vi "Lab Panel V6.00.vi"() -> ()   [LabVIEW 2017] (continued)
                        n2201 = local read "AI data 1"() -> (w3889:waveform(dbl)[])
                        n2202 = local read "AI data 2"() -> (w3886:waveform(dbl)[])
                        n2203 = local read "AI Error"() -> (w3888:errorcluster[])
                        n2204 = call "sub vi - Read Analog All v9.5.vi"("data 0"=w3890, "data 1"=w3889, "data 2"=w3886, "AI Error"=w3888) -> ("Lab05 -1 Offset I"=→"Lab05 -1 Offset I":dbl, "array GRAPH"=w3898:dynamicdata[], "LAB01"=w3897:T33, "LAB02"=w3896:T34, "LAB03"=w3895:T35, "LAB04"=w3894:T36, "deg C"=w3892:dbl, "USB Error"=w3891:bool[], "LAB05"=w3893:T17)  [unwired: 3 in]
                        "LAB05" <- w3893
                        n2205 = local read "AI loop time"() -> (w3887:dbl)
                      }
                    }
                  }
                  frame True {
                    # "simulate"
                    n2206 = local read "ON amps"() -> (w3902:dbl)
                    n2207 = local read "OFF amps"() -> (w3903:dbl)
                    n2208 = local read "VOLTS"() -> (w3906:dbl)
                    n2209 = local read "PF"() -> (w3905:dbl)
                    n2210 = Select(t=w3902, s=w3908, f=w3903) -> (s? t:f=w3907:dbl)
                    n2211 = Bundle("OFF amps"=w3907, "VOLTS"=w3906, "PF"=w3905, "OFF amps"=w3907, "VOLTS"=w3906, "PF"=w3905) -> (w3904:T37)  [unwired: 1 in]
                  }
                }
                n2212 = local read "DAQ Simulate"() -> (w3861:bool)
                n2213 = stacked-sequence {
                  seq-local: [w3912 _ _ _ _ _ _ _] -> [_ _ _ _ _ _ _ _]
                  seq-local: [w3911 _ _ _ _ _ _ _] -> [_ _ _ _ _ _ _ _]
                  seq-local: [w3910 _ _ _ _ _ _ _] -> [_ _ _ _ _ _ _ w4137]
                  tunnel: w3868 -> [_ w3964 _ _ _ _ _ _]
                  tunnel: w3867 -> [_ _ w3997 _ _ _ _ _]
                  tunnel: w3866 -> [_ _ _ w4031 _ _ _ _]
                  tunnel: w3865 -> [_ _ _ _ w4065 _ _ _]
                  tunnel: w3864 -> [_ _ _ _ _ w4099 _ _]
                  tunnel: w3863 -> [_ _ _ _ _ _ w4134 _]
                  tunnel: w3861 -> [_ _ w3996 w4030 w4064 w4098 w4133 w4139]
                  tunnel: T15 {"1  (A) cal"=1.0, "1 (V) cal"=1.0, "1 (PF) cal"=1.0, "1 (TL) cal"=1.0, "1 (TN) cal"=1.0, "2 (A) cal"=1.0, "2 (V) cal"=1.0, "2 (PF) cal"=1.0, "2 (TL) cal"=1.0, "2 (TN) cal"=1.0} ("CAL LAB01") -> [_ _ w3995 w4029 w4063 w4097 w4132 _]
                  tunnel: w3858 -> [_ _ _ _ _ _ _ w4138]
                  tunnel: w3857 -> [w3915 _ _ _ _ _ _ _]
                  tunnel: w3855 -> [_ w3943 _ _ _ _ _ _]
                  frame #0 {
                    # "Count DAQ errors. If greater than 10 do USB reset"
                    n2214 = Index Array(array=w3915, index=2) -> (element=w3910:bool)
                    n2215 = Index Array(array=w3915, index=1) -> (element=w3911:bool)
                    n2216 = Index Array(array=w3915, index=0) -> (element=w3912:bool)
                    n2217 = local write "Error USB #2"(w3910) -> ()
                    n2218 = local write "Error USB #0"(w3912) -> ()
                    n2219 = local write "Error USB #1"(w3911) -> ()
                    n2220 = stacked-sequence {
                      tunnel: w3912 -> [w3919 _ _ _]
                      tunnel: w3911 -> [_ w3924 _ _]
                      tunnel: 0 -> [w3918 w3923 w3928 _]
                      tunnel: w3910 -> [_ _ w3929 _]
                      frame #0 {
                        n2221 = case shown="True" w3919 {
                          tunnel: w3918 -> [w3920 _]
                          frame False {
                            n2222 = local write "Er USB#0"(w3920) -> ()
                          }
                          frame True {
                            n2223 = local read "Er USB#0"() -> (w3922:dbl)
                            n2224 = Increment(x=w3922) -> (x+1=→"Er USB#0":dbl)
                          }
                        }
                      }
                      frame #1 {
                        n2225 = case shown="True" w3924 {
                          tunnel: w3923 -> [w3925 _]
                          frame False {
                            n2226 = local write "Er USB#1"(w3925) -> ()
                          }
                          frame True {
                            n2227 = local read "Er USB#1"() -> (w3927:dbl)
                            n2228 = Increment(x=w3927) -> (x+1=→"Er USB#1":dbl)
                          }
                        }
                      }
                      frame #2 {
                        n2229 = case shown="True" w3929 {
                          tunnel: w3928 -> [w3930 _]
                          frame False {
                            n2230 = local write "Er USB#2"(w3930) -> ()
                          }
                          frame True {
                            n2231 = local read "Er USB#2"() -> (w3932:dbl)
                            n2232 = Increment(x=w3932) -> (x+1=→"Er USB#2":dbl)
                          }
                        }
                      }
                      frame #3 {
                        w3938 = 10
                        n2233 = local read "Er USB#2"() -> (w3939:dbl)
                        n2234 = local read "Er USB#0"() -> (w3941:dbl)
                        n2235 = local read "Er USB#1"() -> (w3940:dbl)
                        n2236 = Greater Or Equal?(x=w3941, y=w3938) -> (x >= y?=w3936:bool)
                        n2237 = Greater Or Equal?(x=w3940, y=w3938) -> (x >= y?=w3935:bool)
                        n2238 = Greater Or Equal?(x=w3939, y=w3938) -> (x >= y?=w3934:bool)
                        n2239 = Or(x=w3936, y=w3935) -> (x .or. y?=w3937:bool)
                        n2240 = Or(x=w3937, y=w3934) -> (x .or. y?=w3933:bool)
                        "Analog error" <- w3933
                        n2241 = case shown="False" w3933 {
                          frame False {
                            n2242 = call "Less Simple Error Handler.vi"("message"="Error count exceeded") -> ()  [unwired: 5 in]
                          }
                          frame True {
                          }
                        }
                      }
                    }
                  }
                  frame #1 {
                    # "display graph data on ADM page"
                    n2243 = local write "AI loop time"(w3943) -> ()
                    n2244 = local write "AI"(TRUE) -> ()
                    n2245 = Index Array(array=w3964, index=6) -> (element=→"LAB04-1 (GRAPH)":dynamicdata)
                    n2246 = Index Array(array=w3964, index=7) -> (element=→"LAB04-2 (GRAPH)":dynamicdata)
                    n2247 = Index Array(array=w3964, index=9) -> (element=→"LAB05-2 (GRAPH)":dynamicdata)
                    n2248 = Index Array(array=w3964, index=8) -> (element=→"LAB05-1 (GRAPH)":dynamicdata)
                    n2249 = Index Array(array=w3964, index=5) -> (element=→"LAB03-2 (GRAPH)":dynamicdata)
                    n2250 = Index Array(array=w3964, index=0) -> (element=→"LAB01-1 (GRAPH)":dynamicdata)
                    n2251 = Index Array(array=w3964, index=1) -> (element=→"LAB01-2 (GRAPH)":dynamicdata)
                    n2252 = Index Array(array=w3964, index=2) -> (element=→"LAB02-1 (GRAPH)":dynamicdata)
                    n2253 = Index Array(array=w3964, index=3) -> (element=→"LAB02-2 (GRAPH)":dynamicdata)
                    n2254 = Index Array(array=w3964, index=4) -> (element=→"LAB03-1 (GRAPH)":dynamicdata)
                  }
                  frame #2 {
                    n2255 = case shown="False" w3996 {
                      tunnel: [w3998 w3999] -> w3994
                      tunnel: w3995 -> [_ w3999]
                      frame False {
                        n2256 = local read "CAL LAB01"() -> (w3998:T15)
                      }
                      frame True {
                      }
                    }
                    n2257 = Unbundle By Name(w3997) -> ("OFF amps"=w3993:dbl, "VOLTS"=w3992:dbl, "PF"=w3991:dbl, "OFF amps"=w3990:dbl, "VOLTS"=w3989:dbl, "PF"=w3988:dbl)
                    n2258 = Unbundle By Name(w3994) -> ("1  (A) cal"=w3987:dbl, "1 (V) cal"=w3986:dbl, "1 (PF) cal"=w3985:dbl, "2 (A) cal"=w3984:dbl, "2 (V) cal"=w3983:dbl, "2 (PF) cal"=w3982:dbl)  [unwired: 4 out]
                    n2259 = Multiply(x=w3993, y=w3987) -> (x*y=w3979:dbl)
                    n2260 = Multiply(x=w3992, y=w3986) -> (x*y=w3978:dbl)
                    n2261 = Multiply(x=w3991, y=w3985) -> (x*y=w3973:dbl)
                    n2262 = Multiply(x=w3990, y=w3984) -> (x*y=w3976:dbl)
                    n2263 = Multiply(x=w3989, y=w3983) -> (x*y=w3975:dbl)
                    n2264 = Multiply(x=w3988, y=w3982) -> (x*y=w3969:dbl)
                    n2265 = local read "SIG LAB01-2"() -> (w3980:T2)
                    n2266 = call "Check for valid PF.vi"("PF In"=w3973, "VOLTS"=w3978, "Current"=w3979) -> ("PF Out"=w3971:dbl, "V Out"=w3972:dbl, "I Out"=w3977:dbl)  [unwired: 6 in]
                    n2267 = call "Check for valid PF.vi"("PF In"=w3969, "VOLTS"=w3975, "Current"=w3976) -> ("PF Out"=w3968:dbl, "V Out"=w3970:dbl, "I Out"=w3974:dbl)  [unwired: 6 in]
                    n2268 = local read "SIG LAB01-1"() -> (w3981:T2)
                    n2269 = Bundle By Name(cluster=w3981, "AMPS"=w3977, "VOLTS"=w3972, "PF"=w3971) -> (w3967:T2)
                    "SIG LAB01-1" <- w3967
                    n2270 = Bundle By Name(cluster=w3980, "AMPS"=w3974, "VOLTS"=w3970, "PF"=w3968) -> (w3966:T2)
                    "SIG LAB01-2" <- w3966
                    n2271 = global write "Global display 1.vi" "SIG LAB01-2"(w3966) -> ()
                    n2272 = global write "Global display 1.vi" "SIG LAB01-1"(w3967) -> ()
                  }
                  frame #3 {
                    n2273 = Unbundle By Name(w4031) -> ("OFF amps"=w4027:dbl, "VOLTS"=w4026:dbl, "PF"=w4025:dbl, "OFF amps"=w4024:dbl, "VOLTS"=w4023:dbl, "PF"=w4022:dbl)
                    n2274 = case shown="True" w4030 {
                      tunnel: [w4032 w4033] -> w4028
                      tunnel: w4029 -> [_ w4033]
                      frame False {
                        n2275 = local read "CAL LAB02"() -> (w4032:T16)
                      }
                      frame True {
                      }
                    }
                    n2276 = Unbundle By Name(w4028) -> ("1  (A) cal"=w4021:dbl, "1 (V) cal"=w4020:dbl, "1 (PF) cal"=w4019:dbl, "2 (A) cal"=w4018:dbl, "2 (V) cal"=w4017:dbl, "2 (PF) cal"=w4016:dbl)  [unwired: 4 out]
                    n2277 = Multiply(x=w4027, y=w4021) -> (x*y=w4012:dbl)
                    n2278 = Multiply(x=w4026, y=w4020) -> (x*y=w4011:dbl)
                    n2279 = Multiply(x=w4025, y=w4019) -> (x*y=w4004:dbl)
                    n2280 = Multiply(x=w4024, y=w4018) -> (x*y=w4009:dbl)
                    n2281 = Multiply(x=w4023, y=w4017) -> (x*y=w4008:dbl)
                    n2282 = Multiply(x=w4022, y=w4016) -> (x*y=w4003:dbl)
                    n2283 = local read "SIG LAB02-2"() -> (w4014:T2)
                    n2284 = call "Check for valid PF.vi"("PF In"=w4004, "VOLTS"=w4011, "Current"=w4012) -> ("PF Out"=w4006:dbl, "V Out"=w4005:dbl, "I Out"=w4010:dbl)  [unwired: 6 in]
                    n2285 = call "Check for valid PF.vi"("PF In"=w4003, "VOLTS"=w4008, "Current"=w4009) -> ("PF Out"=w4001:dbl, "V Out"=w4002:dbl, "I Out"=w4007:dbl)  [unwired: 6 in]
                    n2286 = local read "SIG LAB02-1"() -> (w4015:T2)
                    n2287 = Bundle By Name(cluster=w4015, "AMPS"=w4010, "VOLTS"=w4005, "PF"=w4006) -> (→"SIG LAB02-1" →"SIG LAB02-2":T2)
                    n2288 = Bundle By Name(cluster=w4014, "AMPS"=w4007, "VOLTS"=w4002, "PF"=w4001) -> (w4013:T2)
                    n2289 = local write "SIG LAB02-2"(w4013) -> ()
                    n2290 = global write "Global display 1.vi" "SIG LAB02-2"(w4013) -> ()
                  }
                  frame #4 {
                    n2291 = Unbundle By Name(w4065) -> ("OFF amps"=w4061:dbl, "VOLTS"=w4060:dbl, "PF"=w4059:dbl, "OFF amps"=w4058:dbl, "VOLTS"=w4057:dbl, "PF"=w4056:dbl)
                    n2292 = case shown="False" w4064 {
                      tunnel: [w4066 w4067] -> w4062
                      tunnel: w4063 -> [_ w4067]
                      frame False {
                        n2293 = local read "CAL LAB03"() -> (w4066:T15)
                      }
                      frame True {
                      }
                    }
                    n2294 = Unbundle By Name(w4062) -> ("1  (A) cal"=w4055:dbl, "1 (V) cal"=w4054:dbl, "1 (PF) cal"=w4053:dbl, "2 (A) cal"=w4052:dbl, "2 (V) cal"=w4051:dbl, "2 (PF) cal"=w4050:dbl)  [unwired: 4 out]
                    n2295 = Multiply(x=w4061, y=w4055) -> (x*y=w4047:dbl)
                    n2296 = Multiply(x=w4060, y=w4054) -> (x*y=w4046:dbl)
                    n2297 = Multiply(x=w4059, y=w4053) -> (x*y=w4041:dbl)
                    n2298 = Multiply(x=w4058, y=w4052) -> (x*y=w4044:dbl)
                    n2299 = Multiply(x=w4057, y=w4051) -> (x*y=w4043:dbl)
                    n2300 = Multiply(x=w4056, y=w4050) -> (x*y=w4040:dbl)
                    n2301 = call "Check for valid PF.vi"("PF In"=w4041, "VOLTS"=w4046, "Current"=w4047) -> ("PF Out"=w4036:dbl, "V Out"=w4037:dbl, "I Out"=w4045:dbl)  [unwired: 6 in]
                    n2302 = call "Check for valid PF.vi"("PF In"=w4040, "VOLTS"=w4043, "Current"=w4044) -> ("PF Out"=w4039:dbl, "V Out"=w4038:dbl, "I Out"=w4042:dbl)  [unwired: 6 in]
                    n2303 = local read "SIG LAB03-1"() -> (w4049:T2)
                    n2304 = local read "SIG LAB03-2"() -> (w4048:T2)
                    n2305 = Bundle By Name(cluster=w4049, "AMPS"=w4045, "VOLTS"=w4037, "PF"=w4036) -> (w4035:T2)
                    "SIG LAB03-1" <- w4035
                    n2306 = Bundle By Name(cluster=w4048, "AMPS"=w4042, "VOLTS"=w4038, "PF"=w4039) -> (w4034:T2)
                    "SIG LAB03-2" <- w4034
                    n2307 = global write "Global display 1.vi" "SIG LAB03-1"(w4035) -> ()
                    n2308 = global write "Global display 1.vi" "SIG LAB03-2"(w4034) -> ()
                  }
                  frame #5 {
                    n2309 = case shown="False" w4098 {
                      tunnel: [w4100 w4101] -> w4096
                      tunnel: w4097 -> [_ w4101]
                      frame False {
                        n2310 = local read "CAL LAB04"() -> (w4100:T15)
                      }
                      frame True {
                      }
                    }
                    n2311 = Unbundle By Name(w4099) -> ("OFF amps"=w4095:dbl, "VOLTS"=w4094:dbl, "PF"=w4093:dbl, "OFF amps"=w4092:dbl, "VOLTS"=w4091:dbl, "PF"=w4090:dbl)
                    n2312 = Unbundle By Name(w4096) -> ("1  (A) cal"=w4089:dbl, "1 (V) cal"=w4088:dbl, "1 (PF) cal"=w4087:dbl, "2 (A) cal"=w4086:dbl, "2 (V) cal"=w4085:dbl, "2 (PF) cal"=w4084:dbl)  [unwired: 4 out]
                    n2313 = Multiply(x=w4095, y=w4089) -> (x*y=w4081:dbl)
                    n2314 = Multiply(x=w4094, y=w4088) -> (x*y=w4080:dbl)
                    n2315 = Multiply(x=w4093, y=w4087) -> (x*y=w4071:dbl)
                    n2316 = Multiply(x=w4092, y=w4086) -> (x*y=w4078:dbl)
                    n2317 = Multiply(x=w4091, y=w4085) -> (x*y=w4077:dbl)
                    n2318 = Multiply(x=w4090, y=w4084) -> (x*y=w4070:dbl)
                    n2319 = local read "SIG LAB04-1"() -> (w4083:T2)
                    n2320 = local read "SIG LAB04-2"() -> (w4082:T2)
                    n2321 = call "Check for valid PF.vi"("PF In"=w4071, "VOLTS"=w4080, "Current"=w4081) -> ("PF Out"=w4074:dbl, "V Out"=w4075:dbl, "I Out"=w4079:dbl)  [unwired: 6 in]
                    n2322 = call "Check for valid PF.vi"("PF In"=w4070, "VOLTS"=w4077, "Current"=w4078) -> ("PF Out"=w4072:dbl, "V Out"=w4073:dbl, "I Out"=w4076:dbl)  [unwired: 6 in]
                    n2323 = Bundle By Name(cluster=w4083, "AMPS"=w4079, "VOLTS"=w4075, "PF"=w4074) -> (w4069:T2)
                    "SIG LAB04-1" <- w4069
                    n2324 = Bundle By Name(cluster=w4082, "AMPS"=w4076, "VOLTS"=w4073, "PF"=w4072) -> (w4068:T2)
                    "SIG LAB04-2" <- w4068
                    n2325 = global write "Global display 1.vi" "SIG LAB04-2"(w4068) -> ()
                    n2326 = global write "Global display 1.vi" "SIG LAB04-1"(w4069) -> ()
                  }
                  frame #6 {
                    n2327 = Unbundle By Name(w4134) -> ("OFF amps"=w4105:dbl, "VOLTS"=w4119:dbl, "PF"=w4130:dbl, "OFF amps"=w4104:dbl, "VOLTS"=w4129:dbl, "PF"=w4128:dbl)
                    "x-y" <- w4105
                    "OFF amps 2" <- w4105
                    n2328 = local read "LAB05 (CAL)"() -> (w4108:T15)
                    n2329 = case shown="True" w4133 {
                      tunnel: [w4135 w4136] -> w4131
                      tunnel: w4132 -> [_ _]
                      tunnel: w4108 -> [w4135 w4136]
                      frame False {
                      }
                      frame True {
                        (unwired) T38 {"1  (A) cal"=1.0, "1 (V) cal"=1.0, "1 (PF) cal"=1.0, "1 (TL) cal"=1.0, "1 (TN) cal"=1.0, "2 (A) cal"=1.0, "2 (V) cal"=1.0, "2 (PF) cal"=1.0, "2 (TL) cal"=1.0, "2 (TN) cal"=1.0, "1  (A)Zero Offset"=0.0, "2  (A)Zero Offset 1"=0.0} ("LAB05 (CAL)")
                      }
                    }
                    n2330 = Unbundle By Name(w4131) -> ("1  (A) cal"=w4127:dbl, "1 (V) cal"=w4126:dbl, "1 (PF) cal"=w4125:dbl, "2 (A) cal"=w4124:dbl, "2 (V) cal"=w4123:dbl, "2 (PF) cal"=w4122:dbl)  [unwired: 2 out]
                    n2331 = Multiply(x=w4119, y=w4126) -> (x*y=w4118:dbl)
                    n2332 = Multiply(x=w4130, y=w4125) -> (x*y=w4114:dbl)
                    n2333 = Multiply(x=w4104, y=w4124) -> (x*y=w4103:dbl)
                    n2334 = Multiply(x=w4129, y=w4123) -> (x*y=w4116:dbl)
                    n2335 = Multiply(x=w4128, y=w4122) -> (x*y=w4111:dbl)
                    n2336 = Multiply(x=w4105, y=w4127) -> (x*y=w4102:dbl)
                    "x*y" <- w4102
                    n2337 = local read "SIG LAB05-2"() -> (w4120:T2)
                    n2338 = call "Check for valid PF.vi"("PF In"=w4111, "VOLTS"=w4116, "Current"=w4103) -> ("PF Out"=w4110:dbl, "V Out"=w4109:dbl, "I Out"=w4115:dbl)  [unwired: 6 in]
                    n2339 = call "Check for valid PF.vi"("PF In"=w4114, "VOLTS"=w4118, "Current"=w4102) -> ("PF Out"=w4113:dbl, "V Out"=w4112:dbl, "I Out"=w4117:dbl)  [unwired: 6 in]
                    n2340 = local read "SIG LAB05-1"() -> (w4121:T2)
                    n2341 = Bundle By Name(cluster=w4121, "AMPS"=w4117, "VOLTS"=w4112, "PF"=w4113) -> (w4107:T2)
                    "SIG LAB05-1" <- w4107
                    n2342 = Bundle By Name(cluster=w4120, "AMPS"=w4115, "VOLTS"=w4109, "PF"=w4110) -> (w4106:T2)
                    "SIG LAB05-2" <- w4106
                    n2343 = global write "Global display 1.vi" "SIG LAB05-1"(w4107) -> ()
                    n2344 = global write "Global display 1.vi" "SIG LAB05-2"(w4106) -> ()
                  }
                  frame #7 {
                    n2345 = case shown="False" w4137 {
                      tunnel: w4139 -> [w4144 _]
                      tunnel: w4138 -> [w4143 _]
                      frame False {
                        # "update ambient referance temperature"
                        n2346 = case shown="False" w4144 {
                          tunnel: [w4146 100.0] -> w4145
                          frame False {
                            n2347 = local read "TEMP REF cal"() -> (w4146:dbl)
                          }
                          frame True {
                          }
                        }
                        n2348 = disable-structure shown="Disabled" {
                          frame Disabled {
                            n2349 = local read "Temp read loop"() -> ()  [unwired: 1 out]
                          }
                          frame Enabled {
                          }
                        }
                        n2350 = Multiply(x=w4145, y=w4143) -> (x*y=w4142:dbl)
                        n2351 = Subtract(x=w4142, y=272) -> (x-y=w4140:dbl)
                        "Amb Temp" <- w4140
                        n2352 = local write "Ref deg C"(w4140) -> ()
                        "deg C (volts)" <- w4143
                      }
                      frame True {
                      }
                    }
                  }
                }
              }
            }
          }
          frame #14 {
            # "save test data to file during testing"
            n2353 = local read "on loops"() -> (w4167:dbl)
            n2354 = Get Date/Time In Seconds() -> (seconds since 1Jan1904=w4148:timestamp)
            "File Time Stamp" <- w4148
            n2355 = local read "jig cycle"() -> (w4164:dbl)
            n2356 = Format Date/Time String(time format string (%c)="%H:%M%:%S", seconds (now)=w4148) -> (date/time string=w4152:string)  [unwired: 1 in]
            n2357 = Add(x=w4167, y=4) -> (x+y=w4165:dbl)
            n2358 = Build Array(w4152) -> (w4151:string[])
            n2359 = Equal?(x=w4164, y=3) -> (x = y?=w4150:bool)
            n2360 = Equal?(x=w4164, y=w4165) -> (x = y?=w4149:bool)
            n2361 = stacked-sequence {
              tunnel: w4163 -> [w4173 _ _ _ _ _ _ _ _ _]
              tunnel: w4162 -> [_ w4249 _ _ _ _ _ _ _ _]
              tunnel: w4161 -> [_ _ w4329 _ _ _ _ _ _ _]
              tunnel: w4160 -> [_ _ _ w4409 _ _ _ _ _ _]
              tunnel: w4159 -> [_ _ _ _ w4489 _ _ _ _ _]
              tunnel: w4158 -> [_ _ _ _ _ w4569 _ _ _ _]
              tunnel: w4157 -> [_ _ _ _ _ _ w4649 _ _ _]
              tunnel: w4156 -> [_ _ _ _ _ _ _ w4729 _ _]
              tunnel: w4155 -> [_ _ _ _ _ _ _ _ w4809 _]
              tunnel: w4154 -> [_ _ _ _ _ _ _ _ _ w4889]
              tunnel: w4151 -> [w4172 w4253 w4333 w4413 w4493 w4573 w4653 w4733 w4813 w4893]
              tunnel: w4150 -> [w4171 w4252 w4332 w4412 w4492 w4572 w4652 w4732 w4812 w4892]
              tunnel: w4149 -> [w4170 w4251 w4331 w4411 w4491 w4571 w4651 w4731 w4811 w4891]
              tunnel: w4148 -> [w4169 w4250 w4330 w4410 w4490 w4570 w4650 w4730 w4810 w4890]
              frame #0 {
                n2362 = case shown="True" w4173 {
                  tunnel: w4172 -> [_ w4178]
                  tunnel: w4171 -> [_ w4177]
                  tunnel: w4170 -> [_ w4175]
                  tunnel: w4169 -> [_ w4174]
                  frame False {
                  }
                  frame True {
                    n2363 = local read "SIG LAB01-1"() -> (w4180:T2)
                    n2364 = local read "ON L01-1"() -> (w4176:cluster{"amps":dbl, "volts":dbl, "pf":dbl})
                    n2365 = local read "DISP LAB01-1"() -> (w4179:T4)
                    n2366 = Unbundle(w4180) -> ("AMPS"=w4186:dbl, "VOLTS"=w4184:dbl, "PF"=w4183:dbl, "Tmp Live"=w4182:dbl, "Tmp Neut"=w4185:dbl)
                    n2367 = Unbundle(w4179) -> ("CYCLE"=w4181:dbl)  [unwired: 2 out]
                    n2368 = stacked-sequence {
                      tunnel: w4186 -> [w4190 w4209]
                      tunnel: w4185 -> [_ w4208]
                      tunnel: w4184 -> [w4189 w4207]
                      tunnel: w4183 -> [w4188 w4206]
                      tunnel: w4182 -> [_ w4205]
                      tunnel: w4181 -> [_ w4204]
                      tunnel: w4178 -> [_ w4203]
                      tunnel: w4177 -> [w4191 _]
                      tunnel: w4176 -> [w4187 w4201]
                      tunnel: w4175 -> [_ w4202]
                      tunnel: w4174 -> [_ w4197]
                      frame #0 {
                        n2369 = case shown="True" w4191 {
                          tunnel: w4190 -> [_ w4196]
                          tunnel: w4189 -> [_ w4195]
                          tunnel: w4188 -> [_ w4194]
                          tunnel: w4187 -> [_ w4192]
                          frame False {
                          }
                          frame True {
                            n2370 = Bundle(cluster=w4192, "amps"=w4196, "volts"=w4195, "pf"=w4194) -> (w4193:cluster{"amps":dbl, "volts":dbl, "pf":dbl})
                            n2371 = local write "ON L01-1"(w4193) -> ()
                          }
                        }
                      }
                      frame #1 {
                        n2372 = Unbundle(w4201) -> ("amps"=w4200:dbl, "volts"=w4199:dbl, "pf"=w4198:dbl)
                        n2373 = case shown="True" w4202 {
                          tunnel: w4209 -> [_ w4210]
                          tunnel: w4208 -> [_ w4248]
                          tunnel: w4207 -> [_ _]
                          tunnel: w4206 -> [_ _]
                          tunnel: w4205 -> [_ w4247]
                          tunnel: w4204 -> [_ w4246]
                          tunnel: w4203 -> [_ w4214]
                          tunnel: w4200 -> [_ w4211]
                          tunnel: w4199 -> [_ w4243]
                          tunnel: w4198 -> [_ w4242]
                          tunnel: w4197 -> [_ w4212]
                          frame False {
                          }
                          frame True {
                            n2374 = local read "TDMS LAB01-1"() -> (w4245:refnum<k34>)
                            n2375 = Build Array(w4243) -> (w4239:dbl[])
                            n2376 = Build Array(w4242) -> (w4238:dbl[])
                            n2377 = Build Array(w4247) -> (w4237:dbl[])
                            n2378 = Build Array(w4248) -> (w4236:dbl[])
                            n2379 = Build Array(w4211) -> (w4241:dbl[])
                            n2380 = Build Array(w4210) -> (w4240:dbl[])
                            n2381 = Build Array(w4246) -> (w4235:dbl[])
                            n2382 = Build Array("AMPS ON", "AMPS OFF", "VOLTS", "PF", "TEMP Live", "TEMP Neut", "CYCLE") -> (w4219:string[])
                            n2383 = Bundle By Name("Y"=w4241, "t0"=w4212) -> (w4234:waveform(dbl))  [unwired: 1 in]
                            n2384 = Bundle By Name("Y"=w4240, "t0"=w4212) -> (w4233:waveform(dbl))  [unwired: 1 in]
                            n2385 = Bundle By Name("Y"=w4239, "t0"=w4212) -> (w4232:waveform(dbl))  [unwired: 1 in]
                            n2386 = Bundle By Name("Y"=w4238, "t0"=w4212) -> (w4231:waveform(dbl))  [unwired: 1 in]
                            n2387 = Bundle By Name("Y"=w4237, "t0"=w4212) -> (w4230:waveform(dbl))  [unwired: 1 in]
                            n2388 = Bundle By Name("Y"=w4236, "t0"=w4212) -> (w4229:waveform(dbl))  [unwired: 1 in]
                            n2389 = Bundle By Name("Y"=w4235, "t0"=w4212) -> (w4228:waveform(dbl))  [unwired: 1 in]
                            n2390 = Build Array(w4234, w4233, w4232, w4231, w4230, w4229, w4228) -> (w4227:waveform(dbl)[])
                            n2391 = TDMS Write(0:w4245, 5:"TEST VALUES", 7:w4219, 9:w4227) -> (4:w4218:refnum<k34>, 6:w4217:string, 15:w4216:errorcluster)  [unwired: 2 in, 1 out]
                            n2392 = TDMS Write(0:w4218, 5:w4217, 7:"TIME", 9:w4214, 11:w4216) -> (15:w4213:errorcluster)  [unwired: 1 in, 3 out]
                            n2393 = local write "data file error"(w4213) -> ()
                          }
                        }
                      }
                    }
                  }
                }
              }
              frame #1 {
                n2394 = case shown="True" w4249 {
                  tunnel: w4253 -> [_ w4258]
                  tunnel: w4252 -> [_ w4257]
                  tunnel: w4251 -> [_ w4255]
                  tunnel: w4250 -> [_ w4254]
                  frame False {
                  }
                  frame True {
                    n2395 = local read "DISP LAB01-2"() -> (w4259:T4)
                    n2396 = local read "SIG LAB01-2"() -> (w4260:T2)
                    n2397 = local read "ON L01-2"() -> (w4256:cluster{"amps":dbl, "volts":dbl, "pf":dbl})
                    n2398 = Unbundle(w4260) -> ("AMPS"=w4266:dbl, "VOLTS"=w4264:dbl, "PF"=w4263:dbl, "Tmp Live"=w4262:dbl, "Tmp Neut"=w4265:dbl)
                    n2399 = Unbundle(w4259) -> ("CYCLE"=w4261:dbl)  [unwired: 2 out]
                    n2400 = stacked-sequence {
                      tunnel: w4266 -> [w4270 w4289]
                      tunnel: w4265 -> [_ w4288]
                      tunnel: w4264 -> [w4269 w4287]
                      tunnel: w4263 -> [w4268 w4286]
                      tunnel: w4262 -> [_ w4285]
                      tunnel: w4261 -> [_ w4284]
                      tunnel: w4258 -> [_ w4283]
                      tunnel: w4257 -> [w4271 _]
                      tunnel: w4256 -> [w4267 w4281]
                      tunnel: w4255 -> [_ w4282]
                      tunnel: w4254 -> [_ w4277]
                      frame #0 {
                        n2401 = case shown="True" w4271 {
                          tunnel: w4270 -> [_ w4276]
                          tunnel: w4269 -> [_ w4275]
                          tunnel: w4268 -> [_ w4274]
                          tunnel: w4267 -> [_ w4272]
                          frame False {
                          }
                          frame True {
                            n2402 = Bundle(cluster=w4272, "amps"=w4276, "volts"=w4275, "pf"=w4274) -> (w4273:cluster{"amps":dbl, "volts":dbl, "pf":dbl})
                            n2403 = local write "ON L01-2"(w4273) -> ()
                          }
                        }
                      }
                      frame #1 {
                        n2404 = Unbundle(w4281) -> ("amps"=w4280:dbl, "volts"=w4279:dbl, "pf"=w4278:dbl)
                        n2405 = case shown="True" w4282 {
                          tunnel: w4289 -> [_ w4321]
                          tunnel: w4288 -> [_ w4328]
                          tunnel: w4287 -> [_ _]
                          tunnel: w4286 -> [_ _]
                          tunnel: w4285 -> [_ w4327]
                          tunnel: w4284 -> [_ w4326]
                          tunnel: w4283 -> [_ w4291]
                          tunnel: w4280 -> [_ w4323]
                          tunnel: w4279 -> [_ w4322]
                          tunnel: w4278 -> [_ w4320]
                          tunnel: w4277 -> [_ w4312]
                          frame False {
                          }
                          frame True {
                            n2406 = local read "TDMS LAB01-2"() -> (w4325:refnum<k34>)
                            n2407 = Build Array(w4322) -> (w4317:dbl[])
                            n2408 = Build Array(w4320) -> (w4316:dbl[])
                            n2409 = Build Array(w4327) -> (w4315:dbl[])
                            n2410 = Build Array(w4328) -> (w4314:dbl[])
                            n2411 = Build Array(w4323) -> (w4319:dbl[])
                            n2412 = Build Array(w4321) -> (w4318:dbl[])
                            n2413 = Build Array(w4326) -> (w4313:dbl[])
                            n2414 = Build Array("AMPS ON", "AMPS OFF", "VOLTS", "PF", "TEMP Live", "TEMP Neut", "CYCLE") -> (w4296:string[])
                            n2415 = Bundle By Name("Y"=w4319, "t0"=w4312) -> (w4311:waveform(dbl))  [unwired: 1 in]
                            n2416 = Bundle By Name("Y"=w4318, "t0"=w4312) -> (w4310:waveform(dbl))  [unwired: 1 in]
                            n2417 = Bundle By Name("Y"=w4317, "t0"=w4312) -> (w4309:waveform(dbl))  [unwired: 1 in]
                            n2418 = Bundle By Name("Y"=w4316, "t0"=w4312) -> (w4308:waveform(dbl))  [unwired: 1 in]
                            n2419 = Bundle By Name("Y"=w4315, "t0"=w4312) -> (w4307:waveform(dbl))  [unwired: 1 in]
                            n2420 = Bundle By Name("Y"=w4314, "t0"=w4312) -> (w4306:waveform(dbl))  [unwired: 1 in]
                            n2421 = Bundle By Name("Y"=w4313, "t0"=w4312) -> (w4305:waveform(dbl))  [unwired: 1 in]
                            n2422 = Build Array(w4311, w4310, w4309, w4308, w4307, w4306, w4305) -> (w4304:waveform(dbl)[])
                            n2423 = TDMS Write(0:w4325, 5:"TEST VALUES", 7:w4296, 9:w4304) -> (4:w4295:refnum<k34>, 6:w4294:string, 15:w4293:errorcluster)  [unwired: 2 in, 1 out]
                            n2424 = TDMS Write(0:w4295, 5:w4294, 7:"TIME", 9:w4291, 11:w4293) -> (15:w4290:errorcluster)  [unwired: 1 in, 3 out]
                            n2425 = local write "data file error"(w4290) -> ()
                          }
                        }
                      }
                    }
                  }
                }
              }
              frame #2 {
                n2426 = case shown="True" w4329 {
                  tunnel: w4333 -> [_ w4338]
                  tunnel: w4332 -> [_ w4337]
                  tunnel: w4331 -> [_ w4335]
                  tunnel: w4330 -> [_ w4334]
                  frame False {
                  }
                  frame True {
                    n2427 = local read "DISP LAB02-1"() -> (w4339:T4)
                    n2428 = local read "SIG LAB02-1"() -> (w4340:T2)
                    n2429 = local read "ON L02-1"() -> (w4336:cluster{"amps":dbl, "volts":dbl, "pf":dbl})
                    n2430 = Unbundle(w4340) -> ("AMPS"=w4346:dbl, "VOLTS"=w4344:dbl, "PF"=w4343:dbl, "Tmp Live"=w4342:dbl, "Tmp Neut"=w4345:dbl)
                    n2431 = Unbundle(w4339) -> ("CYCLE"=w4341:dbl)  [unwired: 2 out]
                    n2432 = stacked-sequence {
                      tunnel: w4346 -> [w4350 w4369]
                      tunnel: w4345 -> [_ w4368]
                      tunnel: w4344 -> [w4349 w4367]
                      tunnel: w4343 -> [w4348 w4366]
                      tunnel: w4342 -> [_ w4365]
                      tunnel: w4341 -> [_ w4364]
                      tunnel: w4338 -> [_ w4363]
                      tunnel: w4337 -> [w4351 _]
                      tunnel: w4336 -> [w4347 w4361]
                      tunnel: w4335 -> [_ w4362]
                      tunnel: w4334 -> [_ w4357]
                      frame #0 {
                        n2433 = case shown="True" w4351 {
                          tunnel: w4350 -> [_ w4356]
                          tunnel: w4349 -> [_ w4355]
                          tunnel: w4348 -> [_ w4354]
                          tunnel: w4347 -> [_ w4352]
                          frame False {
                          }
                          frame True {
                            n2434 = Bundle(cluster=w4352, "amps"=w4356, "volts"=w4355, "pf"=w4354) -> (w4353:cluster{"amps":dbl, "volts":dbl, "pf":dbl})
                            n2435 = local write "ON L02-1"(w4353) -> ()
                          }
                        }
                      }
                      frame #1 {
                        n2436 = Unbundle(w4361) -> ("amps"=w4360:dbl, "volts"=w4359:dbl, "pf"=w4358:dbl)
                        n2437 = case shown="True" w4362 {
                          tunnel: w4369 -> [_ w4401]
                          tunnel: w4368 -> [_ w4408]
                          tunnel: w4367 -> [_ _]
                          tunnel: w4366 -> [_ _]
                          tunnel: w4365 -> [_ w4407]
                          tunnel: w4364 -> [_ w4406]
                          tunnel: w4363 -> [_ w4371]
                          tunnel: w4360 -> [_ w4403]
                          tunnel: w4359 -> [_ w4402]
                          tunnel: w4358 -> [_ w4400]
                          tunnel: w4357 -> [_ w4392]
                          frame False {
                          }
                          frame True {
                            n2438 = local read "TDMS LAB02-1"() -> (w4405:refnum<k34>)
                            n2439 = Build Array(w4402) -> (w4397:dbl[])
                            n2440 = Build Array(w4400) -> (w4396:dbl[])
                            n2441 = Build Array(w4407) -> (w4395:dbl[])
                            n2442 = Build Array(w4408) -> (w4394:dbl[])
                            n2443 = Build Array(w4403) -> (w4399:dbl[])
                            n2444 = Build Array(w4401) -> (w4398:dbl[])
                            n2445 = Build Array(w4406) -> (w4393:dbl[])
                            n2446 = Build Array("AMPS ON", "AMPS OFF", "VOLTS", "PF", "TEMP Live", "TEMP Neut", "CYCLE") -> (w4376:string[])
                            n2447 = Bundle By Name("Y"=w4399, "t0"=w4392) -> (w4391:waveform(dbl))  [unwired: 1 in]
                            n2448 = Bundle By Name("Y"=w4398, "t0"=w4392) -> (w4390:waveform(dbl))  [unwired: 1 in]
                            n2449 = Bundle By Name("Y"=w4397, "t0"=w4392) -> (w4389:waveform(dbl))  [unwired: 1 in]
                            n2450 = Bundle By Name("Y"=w4396, "t0"=w4392) -> (w4388:waveform(dbl))  [unwired: 1 in]
                            n2451 = Bundle By Name("Y"=w4395, "t0"=w4392) -> (w4387:waveform(dbl))  [unwired: 1 in]
                            n2452 = Bundle By Name("Y"=w4394, "t0"=w4392) -> (w4386:waveform(dbl))  [unwired: 1 in]
                            n2453 = Bundle By Name("Y"=w4393, "t0"=w4392) -> (w4385:waveform(dbl))  [unwired: 1 in]
                            n2454 = Build Array(w4391, w4390, w4389, w4388, w4387, w4386, w4385) -> (w4384:waveform(dbl)[])
                            n2455 = TDMS Write(0:w4405, 5:"TEST VALUES", 7:w4376, 9:w4384) -> (4:w4375:refnum<k34>, 6:w4374:string, 15:w4373:errorcluster)  [unwired: 2 in, 1 out]
                            n2456 = TDMS Write(0:w4375, 5:w4374, 7:"TIME", 9:w4371, 11:w4373) -> (15:w4370:errorcluster)  [unwired: 1 in, 3 out]
                            n2457 = local write "data file error"(w4370) -> ()
                          }
                        }
                      }
                    }
                  }
                }
              }
              frame #3 {
                n2458 = case shown="True" w4409 {
                  tunnel: w4413 -> [_ w4418]
                  tunnel: w4412 -> [_ w4417]
                  tunnel: w4411 -> [_ w4415]
                  tunnel: w4410 -> [_ w4414]
                  frame False {
                  }
                  frame True {
                    n2459 = local read "DISP LAB02-2"() -> (w4419:T4)
                    n2460 = local read "SIG LAB02-2"() -> (w4420:T2)
                    n2461 = local read "ON L02-2"() -> (w4416:cluster{"amps":dbl, "volts":dbl, "pf":dbl})
                    n2462 = Unbundle(w4420) -> ("AMPS"=w4426:dbl, "VOLTS"=w4424:dbl, "PF"=w4423:dbl, "Tmp Live"=w4422:dbl, "Tmp Neut"=w4425:dbl)
                    n2463 = Unbundle(w4419) -> ("CYCLE"=w4421:dbl)  [unwired: 2 out]
                    n2464 = stacked-sequence {
                      tunnel: w4426 -> [w4430 w4449]
                      tunnel: w4425 -> [_ w4448]
                      tunnel: w4424 -> [w4429 w4447]
                      tunnel: w4423 -> [w4428 w4446]
                      tunnel: w4422 -> [_ w4445]
                      tunnel: w4421 -> [_ w4444]
                      tunnel: w4418 -> [_ w4443]
                      tunnel: w4417 -> [w4431 _]
                      tunnel: w4416 -> [w4427 w4441]
                      tunnel: w4415 -> [_ w4442]
                      tunnel: w4414 -> [_ w4437]
                      frame #0 {
                        n2465 = case shown="True" w4431 {
                          tunnel: w4430 -> [_ w4436]
                          tunnel: w4429 -> [_ w4435]
                          tunnel: w4428 -> [_ w4434]
                          tunnel: w4427 -> [_ w4432]
                          frame False {
                          }
                          frame True {
                            n2466 = Bundle(cluster=w4432, "amps"=w4436, "volts"=w4435, "pf"=w4434) -> (w4433:cluster{"amps":dbl, "volts":dbl, "pf":dbl})
                            n2467 = local write "ON L02-2"(w4433) -> ()
                          }
                        }
                      }
                      frame #1 {
                        n2468 = Unbundle(w4441) -> ("amps"=w4440:dbl, "volts"=w4439:dbl, "pf"=w4438:dbl)
                        n2469 = case shown="True" w4442 {
                          tunnel: w4449 -> [_ w4481]
                          tunnel: w4448 -> [_ w4488]
                          tunnel: w4447 -> [_ _]
                          tunnel: w4446 -> [_ _]
                          tunnel: w4445 -> [_ w4487]
                          tunnel: w4444 -> [_ w4486]
                          tunnel: w4443 -> [_ w4451]
                          tunnel: w4440 -> [_ w4483]
                          tunnel: w4439 -> [_ w4482]
                          tunnel: w4438 -> [_ w4480]
                          tunnel: w4437 -> [_ w4472]
                          frame False {
                          }
                          frame True {
                            n2470 = local read "TDMS LAB02-2"() -> (w4485:refnum<k34>)
                            n2471 = Build Array(w4482) -> (w4477:dbl[])
                            n2472 = Build Array(w4480) -> (w4476:dbl[])
                            n2473 = Build Array(w4487) -> (w4475:dbl[])
                            n2474 = Build Array(w4488) -> (w4474:dbl[])
                            n2475 = Build Array(w4483) -> (w4479:dbl[])
                            n2476 = Build Array(w4481) -> (w4478:dbl[])
                            n2477 = Build Array(w4486) -> (w4473:dbl[])
                            n2478 = Build Array("AMPS ON", "AMPS OFF", "VOLTS", "PF", "TEMP Live", "TEMP Neut", "CYCLE") -> (w4456:string[])
                            n2479 = Bundle By Name("Y"=w4479, "t0"=w4472) -> (w4471:waveform(dbl))  [unwired: 1 in]
                            n2480 = Bundle By Name("Y"=w4478, "t0"=w4472) -> (w4470:waveform(dbl))  [unwired: 1 in]
                            n2481 = Bundle By Name("Y"=w4477, "t0"=w4472) -> (w4469:waveform(dbl))  [unwired: 1 in]
                            n2482 = Bundle By Name("Y"=w4476, "t0"=w4472) -> (w4468:waveform(dbl))  [unwired: 1 in]
                            n2483 = Bundle By Name("Y"=w4475, "t0"=w4472) -> (w4467:waveform(dbl))  [unwired: 1 in]
                            n2484 = Bundle By Name("Y"=w4474, "t0"=w4472) -> (w4466:waveform(dbl))  [unwired: 1 in]
                            n2485 = Bundle By Name("Y"=w4473, "t0"=w4472) -> (w4465:waveform(dbl))  [unwired: 1 in]
                            n2486 = Build Array(w4471, w4470, w4469, w4468, w4467, w4466, w4465) -> (w4464:waveform(dbl)[])
                            n2487 = TDMS Write(0:w4485, 5:"TEST VALUES", 7:w4456, 9:w4464) -> (4:w4455:refnum<k34>, 6:w4454:string, 15:w4453:errorcluster)  [unwired: 2 in, 1 out]
                            n2488 = TDMS Write(0:w4455, 5:w4454, 7:"TIME", 9:w4451, 11:w4453) -> (15:w4450:errorcluster)  [unwired: 1 in, 3 out]
                            n2489 = local write "data file error"(w4450) -> ()
                          }
                        }
                      }
                    }
                  }
                }
              }
              frame #4 {
                n2490 = case shown="True" w4489 {
                  tunnel: w4493 -> [_ w4498]
                  tunnel: w4492 -> [_ w4497]
                  tunnel: w4491 -> [_ w4495]
                  tunnel: w4490 -> [_ w4494]
                  frame False {
                  }
                  frame True {
                    n2491 = local read "DISP LAB03-1"() -> (w4499:T4)
                    n2492 = local read "SIG LAB03-1"() -> (w4500:T2)
                    n2493 = local read "ON L03-1"() -> (w4496:cluster{"amps":dbl, "volts":dbl, "pf":dbl})
                    n2494 = Unbundle(w4500) -> ("AMPS"=w4506:dbl, "VOLTS"=w4504:dbl, "PF"=w4503:dbl, "Tmp Live"=w4502:dbl, "Tmp Neut"=w4505:dbl)
                    n2495 = Unbundle(w4499) -> ("CYCLE"=w4501:dbl)  [unwired: 2 out]
                    n2496 = stacked-sequence {
                      tunnel: w4506 -> [w4510 w4529]
                      tunnel: w4505 -> [_ w4528]
                      tunnel: w4504 -> [w4509 w4527]
                      tunnel: w4503 -> [w4508 w4526]
                      tunnel: w4502 -> [_ w4525]
                      tunnel: w4501 -> [_ w4524]
                      tunnel: w4498 -> [_ w4523]
                      tunnel: w4497 -> [w4511 _]
                      tunnel: w4496 -> [w4507 w4521]
                      tunnel: w4495 -> [_ w4522]
                      tunnel: w4494 -> [_ w4517]
                      frame #0 {
                        n2497 = case shown="True" w4511 {
                          tunnel: w4510 -> [_ w4516]
                          tunnel: w4509 -> [_ w4515]
                          tunnel: w4508 -> [_ w4514]
                          tunnel: w4507 -> [_ w4512]
                          frame False {
                          }
                          frame True {
                            n2498 = Bundle(cluster=w4512, "amps"=w4516, "volts"=w4515, "pf"=w4514) -> (w4513:cluster{"amps":dbl, "volts":dbl, "pf":dbl})
                            n2499 = local write "ON L03-1"(w4513) -> ()
                          }
                        }
                      }
                      frame #1 {
                        n2500 = Unbundle(w4521) -> ("amps"=w4520:dbl, "volts"=w4519:dbl, "pf"=w4518:dbl)
                        n2501 = case shown="True" w4522 {
                          tunnel: w4529 -> [_ w4561]
                          tunnel: w4528 -> [_ w4568]
                          tunnel: w4527 -> [_ _]
                          tunnel: w4526 -> [_ _]
                          tunnel: w4525 -> [_ w4567]
                          tunnel: w4524 -> [_ w4566]
                          tunnel: w4523 -> [_ w4531]
                          tunnel: w4520 -> [_ w4563]
                          tunnel: w4519 -> [_ w4562]
                          tunnel: w4518 -> [_ w4560]
                          tunnel: w4517 -> [_ w4552]
                          frame False {
                          }
                          frame True {
                            n2502 = local read "TDMS LAB03-1"() -> (w4565:refnum<k34>)
                            n2503 = Build Array(w4562) -> (w4557:dbl[])
                            n2504 = Build Array(w4560) -> (w4556:dbl[])
                            n2505 = Build Array(w4567) -> (w4555:dbl[])
                            n2506 = Build Array(w4568) -> (w4554:dbl[])
                            n2507 = Build Array(w4563) -> (w4559:dbl[])
                            n2508 = Build Array(w4561) -> (w4558:dbl[])
                            n2509 = Build Array(w4566) -> (w4553:dbl[])
                            n2510 = Build Array("AMPS ON", "AMPS OFF", "VOLTS", "PF", "TEMP Live", "TEMP Neut", "CYCLE") -> (w4536:string[])
                            n2511 = Bundle By Name("Y"=w4559, "t0"=w4552) -> (w4551:waveform(dbl))  [unwired: 1 in]
                            n2512 = Bundle By Name("Y"=w4558, "t0"=w4552) -> (w4550:waveform(dbl))  [unwired: 1 in]
                            n2513 = Bundle By Name("Y"=w4557, "t0"=w4552) -> (w4549:waveform(dbl))  [unwired: 1 in]
                            n2514 = Bundle By Name("Y"=w4556, "t0"=w4552) -> (w4548:waveform(dbl))  [unwired: 1 in]
                            n2515 = Bundle By Name("Y"=w4555, "t0"=w4552) -> (w4547:waveform(dbl))  [unwired: 1 in]
                            n2516 = Bundle By Name("Y"=w4554, "t0"=w4552) -> (w4546:waveform(dbl))  [unwired: 1 in]
                            n2517 = Bundle By Name("Y"=w4553, "t0"=w4552) -> (w4545:waveform(dbl))  [unwired: 1 in]
                            n2518 = Build Array(w4551, w4550, w4549, w4548, w4547, w4546, w4545) -> (w4544:waveform(dbl)[])
                            n2519 = TDMS Write(0:w4565, 5:"TEST VALUES", 7:w4536, 9:w4544) -> (4:w4535:refnum<k34>, 6:w4534:string, 15:w4533:errorcluster)  [unwired: 2 in, 1 out]
                            n2520 = TDMS Write(0:w4535, 5:w4534, 7:"TIME", 9:w4531, 11:w4533) -> (15:w4530:errorcluster)  [unwired: 1 in, 3 out]
                            n2521 = local write "data file error"(w4530) -> ()
                          }
                        }
                      }
                    }
                  }
                }
              }
              frame #5 {
                n2522 = case shown="True" w4569 {
                  tunnel: w4573 -> [_ w4578]
                  tunnel: w4572 -> [_ w4577]
                  tunnel: w4571 -> [_ w4575]
                  tunnel: w4570 -> [_ w4574]
                  frame False {
                  }
                  frame True {
                    n2523 = local read "DISP LAB03-2"() -> (w4579:T4)
                    n2524 = local read "SIG LAB03-2"() -> (w4580:T2)
                    n2525 = local read "ON L03-2"() -> (w4576:cluster{"amps":dbl, "volts":dbl, "pf":dbl})
                    n2526 = Unbundle(w4580) -> ("AMPS"=w4586:dbl, "VOLTS"=w4584:dbl, "PF"=w4583:dbl, "Tmp Live"=w4582:dbl, "Tmp Neut"=w4585:dbl)
                    n2527 = Unbundle(w4579) -> ("CYCLE"=w4581:dbl)  [unwired: 2 out]
                    n2528 = stacked-sequence {
                      tunnel: w4586 -> [w4590 w4609]
                      tunnel: w4585 -> [_ w4608]
                      tunnel: w4584 -> [w4589 w4607]
                      tunnel: w4583 -> [w4588 w4606]
                      tunnel: w4582 -> [_ w4605]
                      tunnel: w4581 -> [_ w4604]
                      tunnel: w4578 -> [_ w4603]
                      tunnel: w4577 -> [w4591 _]
                      tunnel: w4576 -> [w4587 w4601]
                      tunnel: w4575 -> [_ w4602]
                      tunnel: w4574 -> [_ w4597]
                      frame #0 {
                        n2529 = case shown="True" w4591 {
                          tunnel: w4590 -> [_ w4596]
                          tunnel: w4589 -> [_ w4595]
                          tunnel: w4588 -> [_ w4594]
                          tunnel: w4587 -> [_ w4592]
                          frame False {
                          }
                          frame True {
